vi "Act.vi"(8 "error in (no error)":errorcluster, 9 "VI Refnum in":refnum<vi>, 10 "Flex Msg type":refnum<class "Flex Msg.lvclass">, 11 "Get Refnum in":refnum<class "Get Refnum.lvclass">) -> (0 "error out":errorcluster, 1 "Await user action?":bool, 3 "Get Refnum out":refnum<class "Get Refnum.lvclass">)   [LabVIEW 2020, in "Msg.lvlib" / "Get Refnum.lvclass"]
doc: "This implementation retrieves the This VI refnum and returns it on the Refnum Queue and then awaits triggering of the End occurrance. The VI does not wait for user action."
uses:
  Get Refnum.lvclass
  Flex Msg.lvclass
  Get Refnum.lvclass/Get Refnum.ctl
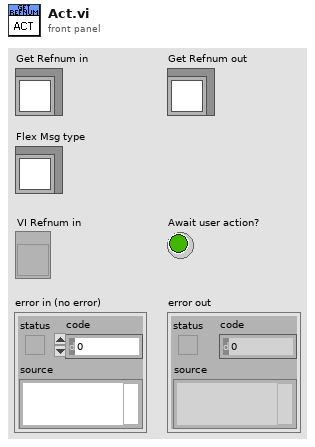
[diagram p1: front panel]
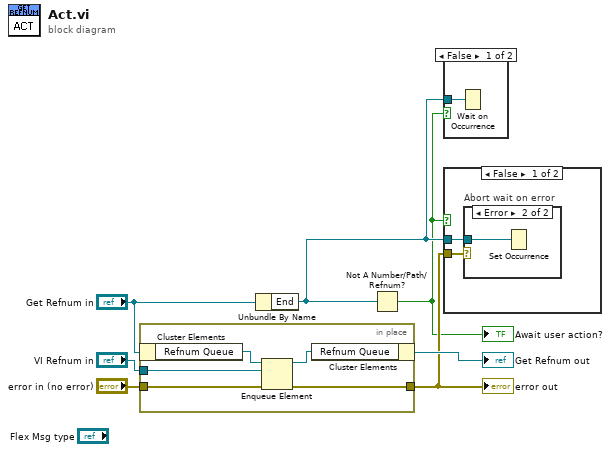
[diagram p0: block diagram]
diagram:
  n1 = in-place {
    in-place-border: "VI Refnum in" -> [w9]
    in-place-border: "error in (no error)" -> [w8]
    in-place-border: [w10] -> w3
    n2 = in-place-cluster #1("Get Refnum in") -> ("Refnum Queue"=w12:refnum<queue>)
    n3 = Enqueue Element(queue=w12, element=w9, error in (no error)=w8) -> (queue out=w11:refnum<queue>, error out=w10:errorcluster)  [unwired: 1 in, 1 out]
    n4 = in-place-cluster #1("Refnum Queue"=w11) -> (→"Get Refnum out":refnum<class "Get Refnum.lvclass">)
  }
  "error out" <- w3
  n5 = Unbundle By Name("Get Refnum in") -> ("End"=w2:refnum<k4>)
  n6 = Not A Number/Path/Refnum?(number/path/refnum=w2) -> (NaN/Path/Refnum?=w1:bool)
  "Await user action?" <- w1
  n7 = case shown="False" w1 {
    tunnel: w2 -> [w13 _]
    frame False {
      n8 = Wait on Occurrence(2:w13) -> ()  [unwired: 2 in, 1 out]
    }
    frame True {
    }
  }
  n9 = case shown="False" w1 {
    tunnel: w3 -> [w15 _]
    tunnel: w2 -> [w14 _]
    frame False {
      n10 = case "Abort wait on error" shown="Error" w15 {
        tunnel: w14 -> [_ w16]
        frame No Error {
        }
        frame Error {
          n11 = Set Occurrence(w16) -> ()
        }
      }
    }
    frame True {
    }
  }
